vi "Populate Single Example Description.vi"(6 "Show FP":bool, 8 "error in (no error)":errorcluster, 10 "VI Description":string, 11 "Path":path) -> (0 "error out":errorcluster)   [LabVIEW 2017, in "csmdoc.lvlib"]
uses:
  csmdoc.lvlib
  _Shared/CSM Shared.lvlib
  _tool/_file/csm-file-support.lvlib
  Communicable State Machine.lvlib
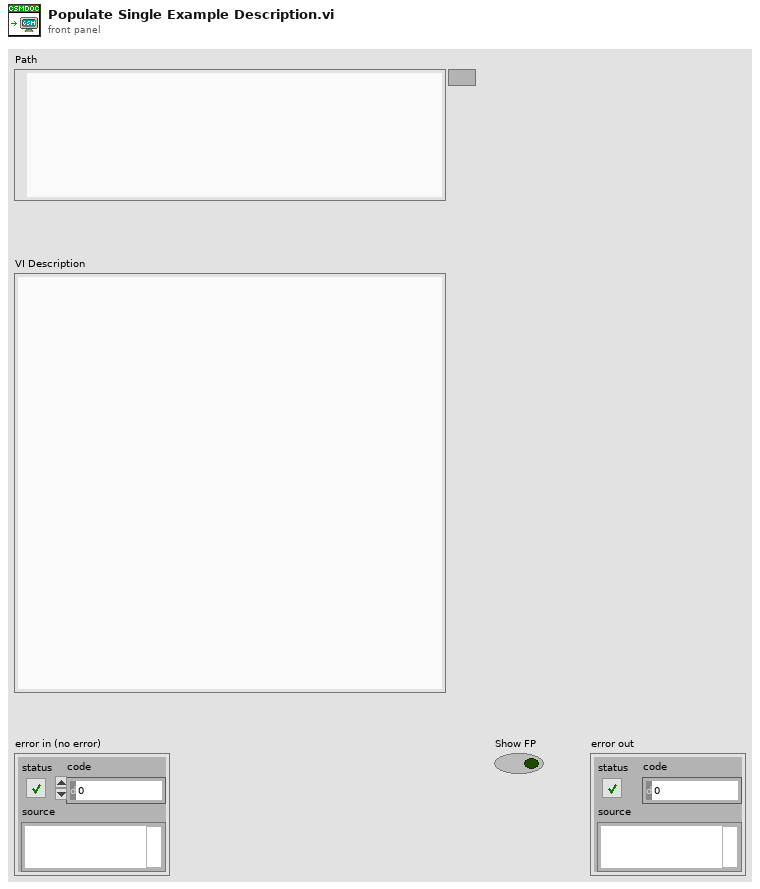
[diagram p1: front panel]
types:
  T1 = typedef "csmdoc.lvlib/DocElement.ctl" = cluster{"ID":string, "Content":string[], "SubIDs":string[], "Path":string[]}
  T2 = typedef "csmdoc.lvlib/DocNote.ctl" = cluster{"ID":string, "Content":string, "Type":string}
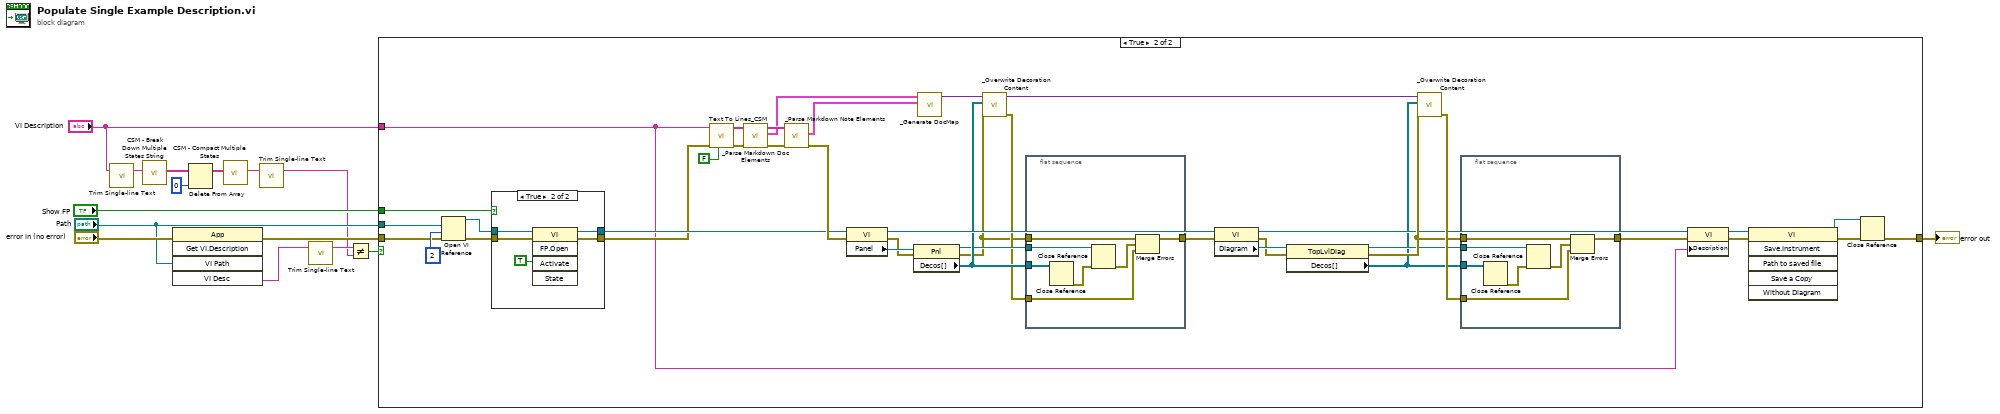
[diagram p0: block diagram]
diagram:
  n1 = call "Trim Single-line Text.vi"("single-line text"="VI Description") -> ("trimed text"=w7:string)  [unwired: 2 in]
  n2 = call "CSM - Break Down Multiple States String.vi"("States"=w7) -> ("Multiple States"=w6:string[])  [unwired: 10 in]
  n3 = invoke class="App" method="Get VI.Description"(error in="error in (no error)", "VI Path"="Path") -> (error out=w15:errorcluster, "VI Desc"=w9:string)  [unwired: 3 in, 3 out]
  n4 = Delete From Array(array=w6, index=0) -> (array with subset deleted=w4:string[])  [unwired: 1 in, 1 out]
  n5 = call "CSM - Compact Multiple States.vi"("Multiple States"=w4) -> ("States"=w3:string)  [unwired: 9 in]
  n6 = call "Trim Single-line Text.vi"("single-line text"=w3) -> ("trimed text"=w1:string)  [unwired: 2 in]
  n7 = call "Trim Single-line Text.vi"("single-line text"=w9) -> ("trimed text"=w13:string)  [unwired: 2 in]
  n8 = Not Equal?(x=w13, y=w1) -> (x != y?=w14:bool)
  n9 = case shown="True" w14 {
    tunnel: w15 -> [w16 w52]
    tunnel: "VI Description" -> [_ w30]
    tunnel: [w16 w49] -> w11
    tunnel: "Show FP" -> [_ w56]
    tunnel: "Path" -> [_ w48]
    frame False {
    }
    frame True {
      n10 = Open VI Reference(vi path=w48, options=2, error in (no error)=w52) -> (vi reference=w53:refnum<vi>, error out=w54:errorcluster)  [unwired: 3 in]
      n11 = case shown="True" w56 {
        tunnel: w54 -> [w71 w76]
        tunnel: w53 -> [w72 w75]
        tunnel: [w71 w74] -> w31
        tunnel: [w72 w73] -> w32
        frame False {
        }
        frame True {
          n12 = invoke class="VI" method="FP.Open"(reference=w75, error in=w76, "Activate"=TRUE ("Activate?")) -> (reference out=w73:refnum<vi>, error out=w74:errorcluster)  [unwired: 2 in, 3 out]
        }
      }
      n13 = call "Text To Lines_CSM.vi"("Remove Empty Lines? (T)"=FALSE ("Remove Empty Lines?(T)"), "error in (no error)"=w31, "String"=w30) -> ("error out"=w45:errorcluster, "Lines"=w46:string[])  [unwired: 7 in]
      n14 = call "_Parse Markdown Doc Elements.vi"("Error in"=w45, "Lines"=w46) -> ("Error out"=w41:errorcluster, "Array"=w39:T1[], "Lines (dup)"=w42:string[])  [unwired: 7 in]
      n15 = call "_Parse Markdown Note Elements.vi"("Error in"=w41, "Lines"=w42) -> ("Error out"=w40:errorcluster, "Array"=w38:T2[])  [unwired: 7 in, 1 out]
      n16 = property class="VI"(reference=w32, error in=w40) -> (reference out=w43:refnum<vi>, error out=w34:errorcluster, "Panel"=w44:refnum<vi>)
      n17 = property class="Pnl"(reference=w44, error in=w34) -> (reference out=w36:refnum<vi>, error out=w28:errorcluster, "Decos[]"=w37:refnum<vi>[])
      n18 = call "_Generate DocMap.vi"("Array 2"=w38, "Array"=w39) -> ("Variant"=w33:variant)  [unwired: 9 in]
      n19 = call "_Overwrite Decoration Content.vi"("error in (no error)"=w28, "Decos[]"=w37, "Variant in"=w33) -> ("error out"=w29:errorcluster, "Variant out"=w22:variant)  [unwired: 7 in]
      n20 = flat-sequence {
        tunnel: w37 -> [w70]
        tunnel: w36 -> [w69]
        tunnel: [w67] -> w35
        tunnel: w28 -> [w65]
        tunnel: w29 -> [w64]
        frame #0 {
          n21 = Close Reference(reference=w70) -> (error out=w68:errorcluster)  [unwired: 1 in]
          n22 = Close Reference(reference=w69, error in (no error)=w68) -> (error out=w66:errorcluster)
          n23 = Merge Errors(w65, w66, w64) -> (w67:errorcluster)
        }
      }
      n24 = property class="VI"(reference=w43, error in=w35) -> (reference out=w21:refnum<vi>, error out=w26:errorcluster, "Diagram"=w27:refnum<vi>)
      n25 = property class="TopLvlDiag"(reference=w27, error in=w26) -> (reference out=w23:refnum<vi>, error out=w24:errorcluster, "Decos[]"=w19:refnum<vi>[])
      n26 = call "_Overwrite Decoration Content.vi"("error in (no error)"=w24, "Decos[]"=w19, "Variant in"=w22) -> ("error out"=w25:errorcluster)  [unwired: 7 in, 1 out]
      n27 = flat-sequence {
        tunnel: w19 -> [w63]
        tunnel: w23 -> [w62]
        tunnel: [w60] -> w20
        tunnel: w24 -> [w58]
        tunnel: w25 -> [w57]
        frame #0 {
          n28 = Close Reference(reference=w63) -> (error out=w61:errorcluster)  [unwired: 1 in]
          n29 = Close Reference(reference=w62, error in (no error)=w61) -> (error out=w59:errorcluster)
          n30 = Merge Errors(w58, w59, w57) -> (w60:errorcluster)
        }
      }
      n31 = property class="VI"(reference=w21, error in=w20, "Description"=w30) -> (reference out=w17:refnum<vi>, error out=w18:errorcluster)
      n32 = invoke class="VI" method="Save.Instrument"(reference=w17, error in=w18) -> (reference out=w50:refnum<vi>, error out=w51:errorcluster)  [unwired: 4 in, 4 out]
      n33 = Close Reference(reference=w50, error in (no error)=w51) -> (error out=w49:errorcluster)
    }
  }
  "error out" <- w11
